vi "Prove Pilot.vi"(7 "Log File Refnum in":refnum<file>, 8 "error in":errorcluster, 9 "Flame Threshold":u32, 10 "Notifiers in":T1, 11 "Boiler Queue in":refnum<queue>) -> (0 "error out":errorcluster, 2 "Notifiers out":T1, 3 "Boiler Queue out":refnum<queue>, 5 "Log File Refnum out":refnum<file>)   [LabVIEW 2017, in "Controller.lvlib"]
doc: "Prove that the pilot light is functioning properly before proceeding."
uses:
  Controller.lvlib
  support/Notifieres/Notifiers.ctl
  support/Message Queue/Message Cluster.ctl
  support/Boiler System Globals.vi
  support/Message Queue/Message Queue.lvlib
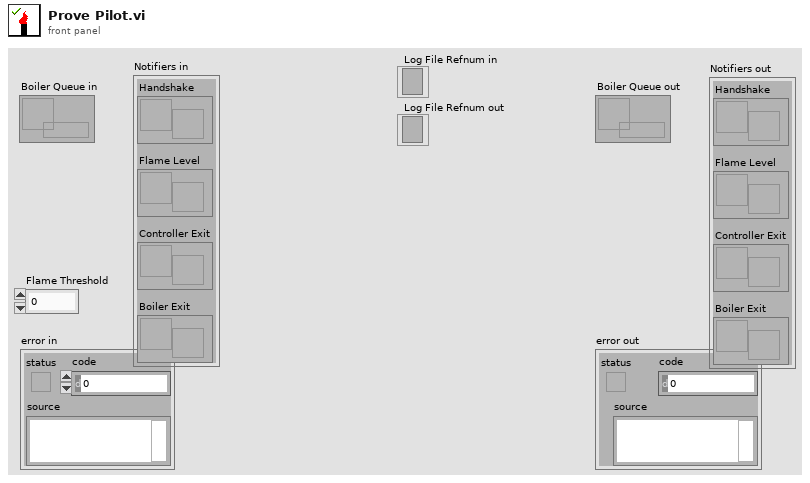
[diagram p1: front panel]
types:
  T1 = typedef "Notifiers.ctl" = cluster{"Handshake":refnum<notifier>, "Flame Level":refnum<notifier>, "Controller Exit":refnum<notifier>, "Boiler Exit":refnum<notifier>}
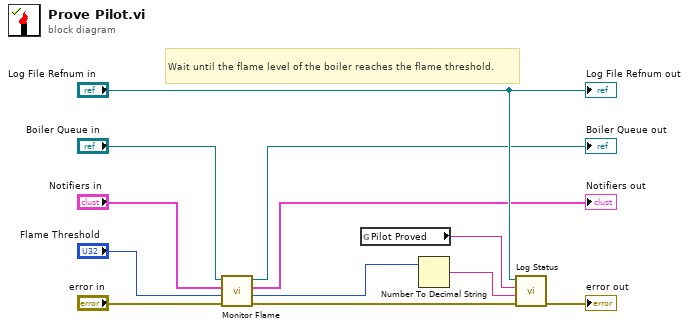
[diagram p0: block diagram]
diagram:
  # "Wait until the flame level of the boiler reaches the flame threshold."
  n1 = call "Monitor Flame.vi"("error in"="error in", "Flame Threshold"="Flame Threshold", "Notifiers in"="Notifiers in", "Boiler Queue in"="Boiler Queue in") -> ("error out"=w5:errorcluster, "Flame Level"=w3:u32, "Notifiers out"=→"Notifiers out":T1, "Boiler Queue out"=→"Boiler Queue out":refnum<queue>)  [unwired: 4 in]
  n2 = global read "Boiler System Globals.vi" "Pilot Proved"() -> (w8:string)
  n3 = Number To Decimal String(number=w3) -> (decimal integer string=w9:string)  [unwired: 1 in]
  n4 = call "Log Status.vi"("error in"=w5, "Event Data String (-)"=w9, "Event String"=w8, "Log File Refnum In"="Log File Refnum in") -> ("error out"=→"error out":errorcluster)  [unwired: 6 in, 1 out]
  "Log File Refnum out" <- "Log File Refnum in"
